vi "STM Comm Lookup Table_Actions.vi"(0 "vi reference":T1, 5 "Connection In":T2, 7 "Index":i32, 9 "Method":T5, 11 "error in (no error)":errorcluster, 12 "Properties out":T4) -> (3 "All Properties":T4[](array[typedef]), 4 "vi reference":T1, 6 "Connection Out":T2, 8 "All Connections":T2[](array[typedef]), 10 "Number of Connections":i32, 14 "Properties out":T4, 15 "error out":errorcluster {"code" min=0 max=0})   [LabVIEW 2015, in "Control Addon Engine.lvlib" / "STM.lvlib"]
uses:
  STM.lvlib
  STM Comm Lookup Table_Ref.ctl
  <vilib>/NI/STM/compatibility/stm_TCPConnectionMethod.ctl
  <vilib>/NI/STM/compatibility/stm_TCP Connection Info.ctl
  <vilib>/NI/STM/compatibility/stm_MetaDataElement.ctl
  <vilib>/NI/STM/compatibility/stm_TCPConnectionProperties.ctl
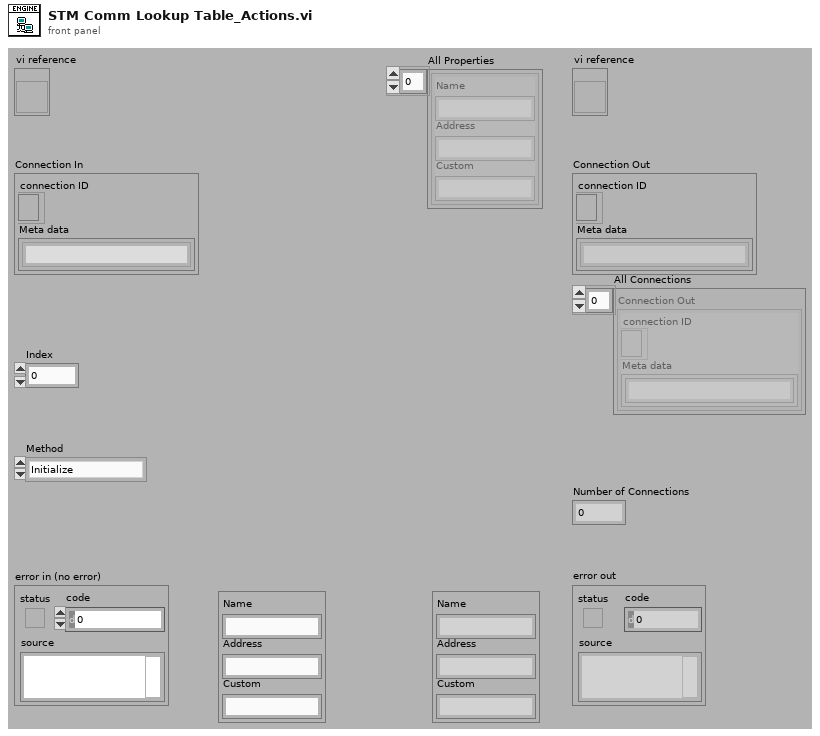
[diagram p1: front panel]
types:
  T1 = typedef "Control Addon Engine.lvlib/STM.lvlib/STM Comm Lookup Table_Ref.ctl" = refnum<vi>
  T2 = typedef "stm_TCP Connection Info.ctl" = cluster{"connection ID":refnum<k5>, "Meta data":T3[]}
  T3 = typedef "stm_MetaDataElement.ctl" = string
  T4 = typedef "stm_TCPConnectionProperties.ctl" = cluster{"Name":string, "Address":string, "Custom":string}
  T5 = typedef "stm_TCPConnectionMethod.ctl" = enum16{"Initialize", "Add Connection", "Set Properties", "Get Connection(s)", "Remove Connection", "Remove All Connections", "Get Connection Count"}
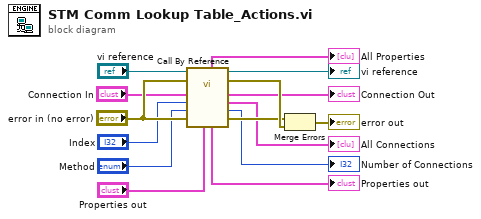
[diagram p0: block diagram]
diagram:
  n1 = call-by-ref "?"(reference="vi reference", error in="error in (no error)", "Properties In"="Properties out", 8:"error in (no error)"="error in (no error)", "Method"="Method", "Index"="Index", "Connection In"="Connection In") -> (reference out=→"vi reference":T1, error out=w14:errorcluster, 0:"error out"=w11:errorcluster, "Number of Connections"=→"Number of Connections":i32, "All Connections"=→"All Connections":T2[], "Connection Out"=→"Connection Out":T2, "Properties out"=→"Properties out":T4, "All Properties"=→"All Properties":T4[])  [unwired: 1 in]
  n2 = Merge Errors(w11, w14) -> (→"error out":errorcluster)
